vi "Simple UDP - Sender2.vi"() -> ()   [LabVIEW 2013]
doc: "The UDP protocol differs from TCP in that there is no error-checking with the packets of information that are sent, and thus no guarantee whatsoever that an intended recipient will actually receive a given piece of data.\n\nUDP does offer the ability to \"broadcast\" data across a network--simply specify an IP Address of all ones (255.255.255.255) to attempt to broadcast information network-wide. Keep in mind that routers and other network hardware will generally refuse to forward the broadcast beyond certain points, so the extent of the broadcast will in practice be limited."
panel:
  out "Current Data Value":u16
  in  "Stop":bool
  # "Overview: Demonstrates the use of the UDP functions to send data over a UDP connection.\nInstructions:\n1. Run the VI.\n2. Open Simple UDP - Receiver.vi and follow the instructions on its front panel.\n3. Click Stop to stop the VI."
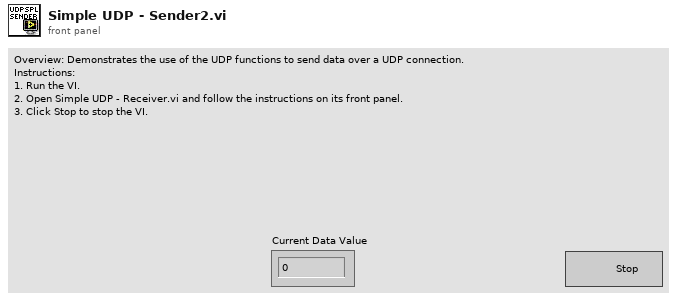
[diagram p1: front panel]
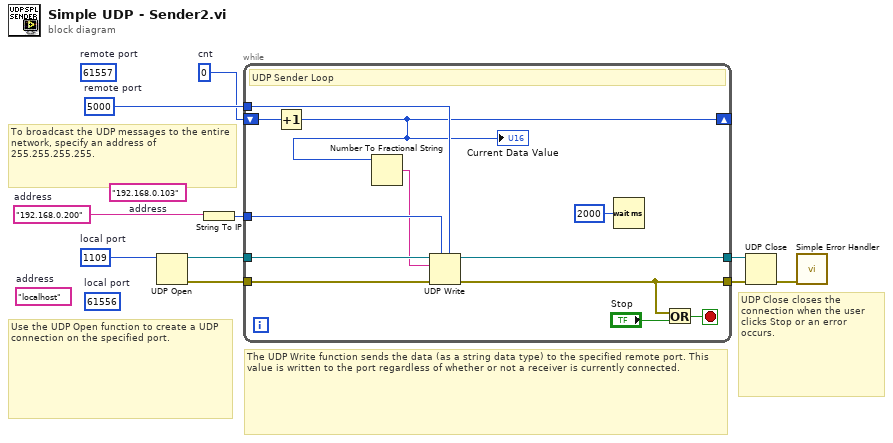
[diagram p0: block diagram]
diagram:
  (unwired) "192.168.0.103"  # address
  w2 = u16 0  # cnt
  (unwired) u16 61557  # remote port
  (unwired) u16 61556  # local port
  w1 = "192.168.0.200"  # address
  w3 = u16 5000  # remote port
  w4 = u16 1109  # local port
  (unwired) "localhost"  # address
  # "To broadcast the UDP messages to the entire network, specify an address of 255.255.255.255."
  # "UDP Close closes the connection when the user clicks Stop or an error occurs."
  # "The UDP Write function sends the data (as a string data type) to the specified remote port. This value is written to the port regardless of whether or not a receiver is currently connected."
  # "Use the UDP Open function to create a UDP connection on the specified port."
  n1 = UDP Open(11:w4) -> (port=w6:refnum<k16>, 0:w5:errorcluster)  [unwired: 4 in, 1 out]
  n2 = String To IP(1:w1) -> (0:w7:u32)
  n3 = while {
    tunnel: [w17] -> w9
    tunnel: w6 -> [w22]
    tunnel: w5 -> [w21]
    tunnel: [w18] -> w10
    tunnel: w7 -> [w16]
    tunnel: w3 -> [w13]
    shift-right: [w11] -> _
    shift-left: w2 -> [w12]
    stop <- w20 stop-if-true
    # "UDP Sender Loop"
    n4 = Increment(x=w12) -> (x+1=w11:u16)
    "Current Data Value" <- w11
    n5 = Number To Fractional String(number=w11) -> (F-format string=w14:string)  [unwired: 3 in]
    n6 = UDP Write(address=w16, port or service name=w13, connection ID=w22, data in=w14, 8:w21) -> (error out=w17:errorcluster, 3:w18:refnum<k16>)  [unwired: 1 in]
    n7 = Wait (ms)(milliseconds to wait=u32 2000) -> ()  [unwired: 1 out]
    n8 = Or(x=w17, y="Stop") -> (x .or. y?=w20:bool)
  }
  n9 = UDP Close(connection ID=w10, 8:w9) -> (error out=w8:errorcluster)  [unwired: 1 out]
  n10 = call <vilib>:"Simple Error Handler.vi"("error in (no error)"=w8) -> ()  [unwired: 4 in, 5 out]
